vi "Address.vi"(10 "NewVal":string, 11 ".NET 참조 번호 입력":refnum<k24>) -> (0 "에러 출력":errorcluster, 3 ".NET 참조 번호 출력":refnum<k24>)   [LabVIEW 2017, in "Retrieved Data.lvclass"]
uses:
  Retrieved Data.lvclass
  C:/Users/KimYG/Application/Solution Package/Minhee Retriever/binaries/Microsoft.WindowsAPICodePack.Shell.dll
  binaries/Microsoft.WindowsAPICodePack.Shell.dll
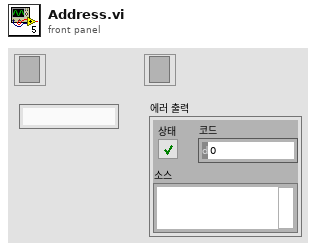
[diagram p1: front panel]
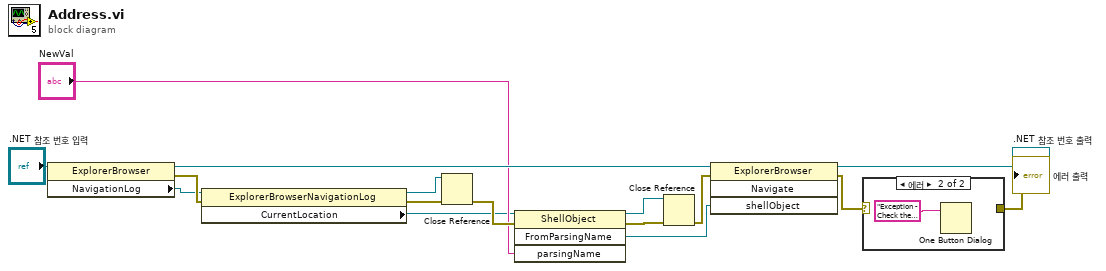
[diagram p0: block diagram]
diagram:
  n1 = property class="ExplorerBrowser"(reference=".NET 참조 번호 입력") -> (reference out=w7:refnum<k24>, error out=w5:errorcluster, "NavigationLog"=w2:refnum<k24>)  [unwired: 1 in]
  n2 = property class="ExplorerBrowserNavigationLog"(reference=w2, error in=w5) -> (reference out=w11:refnum<k24>, error out=w12:errorcluster, "CurrentLocation"=w3:refnum<k24>)
  n3 = Close Reference(reference=w11, error in (no error)=w12) -> (error out=w13:errorcluster)
  n4 = invoke class="ShellObject" method="FromParsingName"(reference=w3, error in=w13, "parsingName"="NewVal") -> (reference out=w8:refnum<k24>, error out=w9:errorcluster, "FromParsingName"=w6:refnum<k24>)  [unwired: 1 in, 1 out]
  n5 = Close Reference(reference=w8, error in (no error)=w9) -> (error out=w10:errorcluster)
  n6 = invoke class="ExplorerBrowser" method="Navigate"(reference=w7, error in=w10, "shellObject"=w6) -> (reference out=→".NET 참조 번호 출력":refnum<k24>, error out=w15:errorcluster)  [unwired: 1 in, 2 out]
  n7 = case shown="에러" w15 {
    selector: w15 -> [w17 _]
    tunnel: [w17 _] -> w16
    frame No Error {
    }
    frame Error {
      n8 = One Button Dialog(message="Exception - Check the navigation address.") -> ()  [unwired: 1 in, 1 out]
    }
  }
  "에러 출력" <- w16
